vi "PathToINIBroadcast.vi"(8 "error in (no error)":errorcluster, 10 "PathToINI":path, 11 "ModuleID":i32) -> (0 "error out":errorcluster)   [LabVIEW 2018, in "AcPwrPlugins.lvlib" / "AcPwrBase.lvclass"]
doc: "This VI brodcast the file explorer location of the INI file that was used to load the plugin."
uses:
  AcPwrBase.lvclass
  clEventType.ctl
  <vilib>/Utility/error.llb/Error Cluster From Error Code.vi
  <vilib>/ErrorRing/Error Ring.xnode
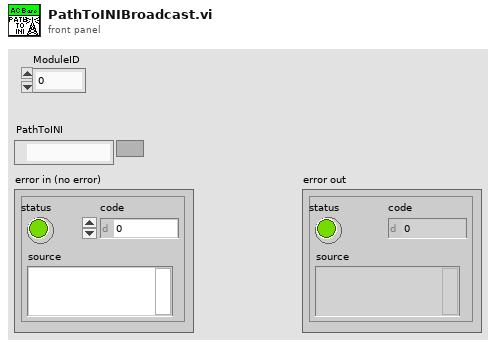
[diagram p1: front panel]
types:
  T1 = typedef "clBroadcastEvents.ctl" = cluster{"DidInit":refnum<user-event>, "StatusUpdate":refnum<user-event>, "ErrorReport":refnum<user-event>, "DidStop":refnum<user-event>, "PathToINI":refnum<user-event>, "Measurements":refnum<user-event>, "LoadConfigFile":refnum<user-event>, "GetSettings":refnum<user-event>, "SetSettings":refnum<user-event>, "GetType&ID":refnum<user-event>, "GotSettings":refnum<user-event>}
  T2 = typedef "clEventType.ctl" = cluster{"ModuleID":i32, "Data":variant}
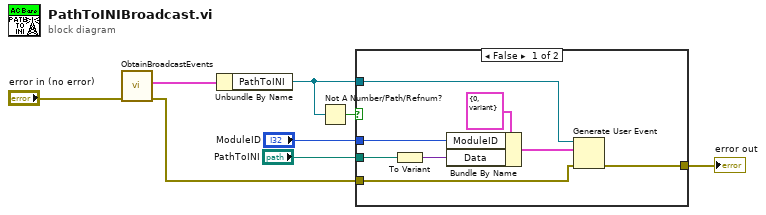
[diagram p0: block diagram]
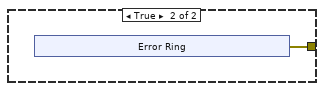
[diagram p2: hidden frame]
diagram:
  n1 = call "ObtainBroadcastEvents.vi"("error in (no error)"="error in (no error)") -> ("error out"=w1:errorcluster, "clAcPwrEvents"=w8:T1)  [unwired: 9 in]
  n2 = Unbundle By Name(w8) -> ("PathToINI"=w4:refnum<user-event>)
  n3 = Not A Number/Path/Refnum?(number/path/refnum=w4) -> (NaN/Path/Refnum?=w5:bool)
  n4 = case shown="False" w5 {
    tunnel: "ModuleID" -> [w15 _]
    tunnel: "PathToINI" -> [w13 _]
    tunnel: w4 -> [w11 _]
    tunnel: [w10 w17] -> w2
    tunnel: w1 -> [w9 _]
    frame False {
      n5 = To Variant(anything=w13) -> (Variant=w14:variant)
      n6 = Bundle By Name(cluster=T2 {"ModuleID"=0, "Data"=variant} ("clEventType"), "ModuleID"=w15, "Data"=w14) -> (w12:T2)
      n7 = Generate User Event(user event=w11, event data cluster=w12, error in=w9) -> (error out=w10:errorcluster)  [unwired: 1 in, 1 out]
    }
    frame True {
      n8 = xnode "Error Ring"() -> ("error out"=w17:errorcluster)
    }
  }
  "error out" <- w2
